vi "version.vi"(8 "error in (no error)":errorcluster) -> (0 "error out":errorcluster, 3 "version":string="1.0.0")   [LabVIEW 2015, in "lv-hello-world.lvlib"]
uses:
  lv-hello-world.lvlib
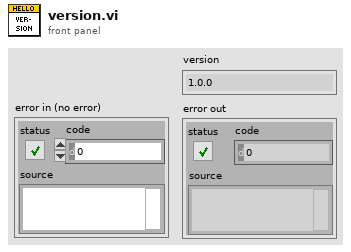
[diagram p1: front panel]
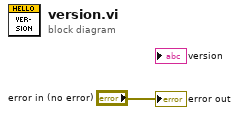
[diagram p0: block diagram]
diagram:
  "error out" <- "error in (no error)"
